vi "Test.vi"() -> ()   [LabVIEW 2015]
uses:
  <vilib>/FPGAPlugInAG/PXIe-7971R/niLvFpga_Open_PXIe-7971R.vi
  <vilib>/Utility/error.llb/Error Cluster From Error Code.vi
  Program Files (x86)/National Instruments/LabVIEW 2015/Targets/NI/FPGA/StockFPGA_IntfPrivate/ScriptTemplates/StockFPGA_PlugInRead32.vi
  <vilib>/rvi/errors/niLvFpgaAdjustHostInterfaceError.vi
  <vilib>/FPGAPlugInAG/PXIe-7971R/niLvFpga_Close_PXIe-7971R.vi
  <vilib>/rvi/interface/nirviOpenFPGA/nirviOpenFPGA.xnode
  FPGA Bitfiles/FPGATesting_FPGATarget_testout_5AUZYZbWs28.lvbitx
  <vilib>/rvi/interface/nirviReadWriteControl/nirviReadWriteControl.xnode
  <vilib>/rvi/interface/nirviCloseFPGA/nirviCloseFPGA.xnode
  <vilib>/FPGAPlugInAG/PXIe-7971R/niLvFpga_Read32_PXIe-7971R.vi
  <vilib>/rvi/interface/nirviReadWriteControl/niFpgaRWControlAccessTimeoutTemplate.vi
  NiFpgaLv.dll
panel:
  out "IO Module\\AI 0":i16
  out "IO Module\\AI 1":i16
  in  "Stop":bool
  in  "DIO 0":u8
  in  "DIO 1":u8
  in  "PFI 3":bool
  in  "PFI 2":bool
  in  "PFI 1":bool
  in  "PFI 0":bool
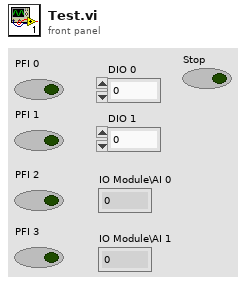
[diagram p1: front panel]
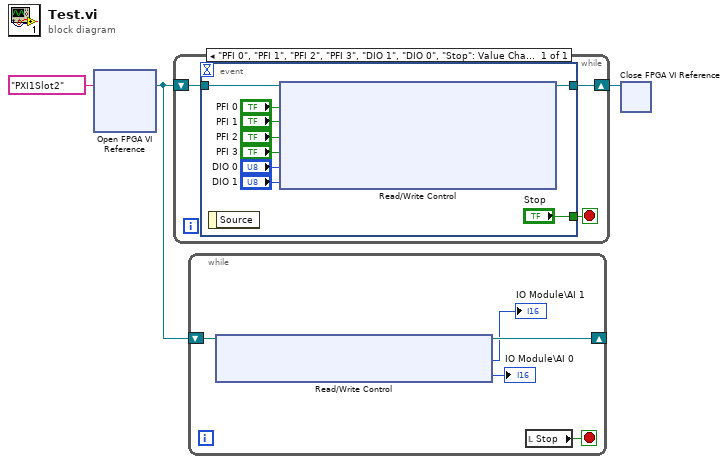
[diagram p0: block diagram]
diagram:
  n1 = xnode "Open FPGA VI Reference"("resource name"=tag "PXI1Slot2") -> ("FPGA VI Reference Out"=w1:refnum<k20>)  [unwired: 1 in, 1 out]
  n2 = while {
    shift-right: [w6] -> w2
    shift-left: w1 -> [w5]
    stop <- w4 stop-if-true
    n3 = event shown="[0] \"PFI 0\", \"PFI 1\", \"PFI 2\", \"PFI 3\", \"DIO 1\", \"DIO 0\", \"Stop\": Value Change" {
      selector: _ -> [_]
      dyn-events: _ -> [_]
      timeout: _ -> [_]
      tunnel: [w15] -> w6
      tunnel: w5 -> [w14]
      tunnel: ["Stop"] -> w4
      event "PFI 0", "PFI 1", "PFI 2", "PFI 3", "DIO 1", "DIO 0", "Stop": Value Change {
        n4 = event-data() -> ()  [unwired: 1 in, 1 out]
        n5 = xnode "Read/Write Control"("FPGA VI Reference In"=w14, "PFI 0"="PFI 0", "PFI 1"="PFI 1", "PFI 2"="PFI 2", "PFI 3"="PFI 3", "DIO 0"="DIO 0", "DIO 1"="DIO 1") -> ("FPGA VI Reference Out"=w15:refnum<k20>)  [unwired: 1 in, 1 out]
      }
    }
  }
  n6 = while {
    shift-right: [w18] -> _
    shift-left: w1 -> [w19]
    stop <- w20 stop-if-true
    n7 = xnode "Read/Write Control"("FPGA VI Reference In"=w19) -> ("FPGA VI Reference Out"=w18:refnum<k20>, "IO Module\\AI 1"=→"IO Module\\AI 1":i16, "IO Module\\AI 0"=→"IO Module\\AI 0":i16)  [unwired: 1 in, 1 out]
    n8 = local read "Stop"() -> (w20:bool)
  }
  n9 = xnode "Close FPGA VI Reference"("FPGA VI Reference In"=w2) -> ()  [unwired: 1 in, 1 out]
